vi "test_MonoMoveAndGetSlitPositionInMM.vi"(0 "device selection":enum16{"monochromator", "CCD", "SCD"}(ring), 1 "Test should pass":bool=TRUE, 5 "set-up a connection":bool=TRUE, 9 "tear down connection":bool=TRUE, 11 "error in":errorcluster, 12 "Delay between send and receive [ms]":i32=100, 13 "wait for procedure to be finished [ms]":i32=4000) -> (10 "log-file path":path, 15 "error out":errorcluster)   [LabVIEW 2023]
uses:
  Classes/Mono/Monochromator.lvclass
  <vilib>/addons/_JKI Toolkits/Caraya/classes/Assert/Assert Equal Value and Type_Variant.vi
  <vilib>/addons/_JKI Toolkits/Caraya/classes/Assert/Assert Not Error.vi
  <vilib>/addons/_JKI Toolkits/Caraya/classes/Test/Test.lvclass
  <vilib>/addons/_JKI Toolkits/Caraya/classes/Assert/Assert.lvclass
  <vilib>/Hampel Software Engineering/HSE Logger/hse-logger.lvlib
panel:
  out "device is open?":bool
  # "Connector Pane"
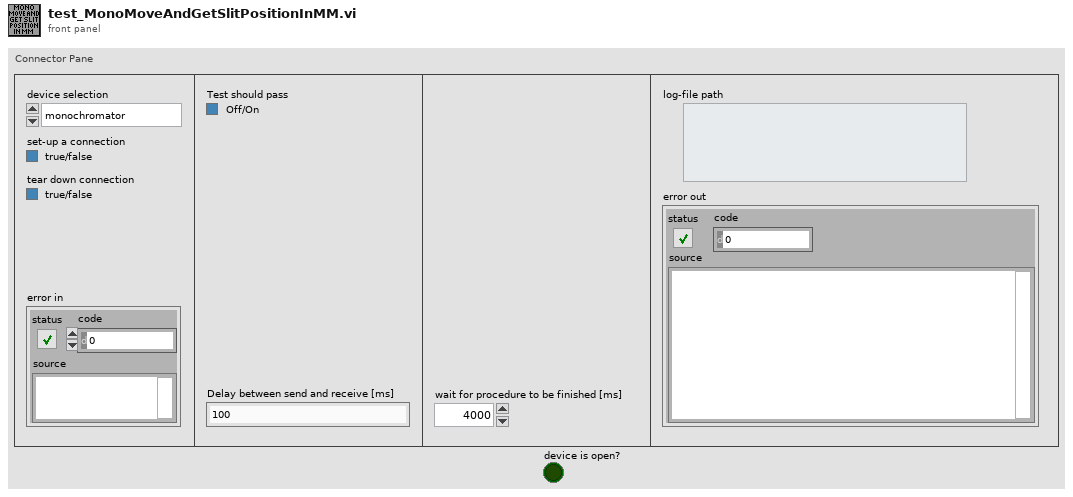
[diagram p1: front panel]
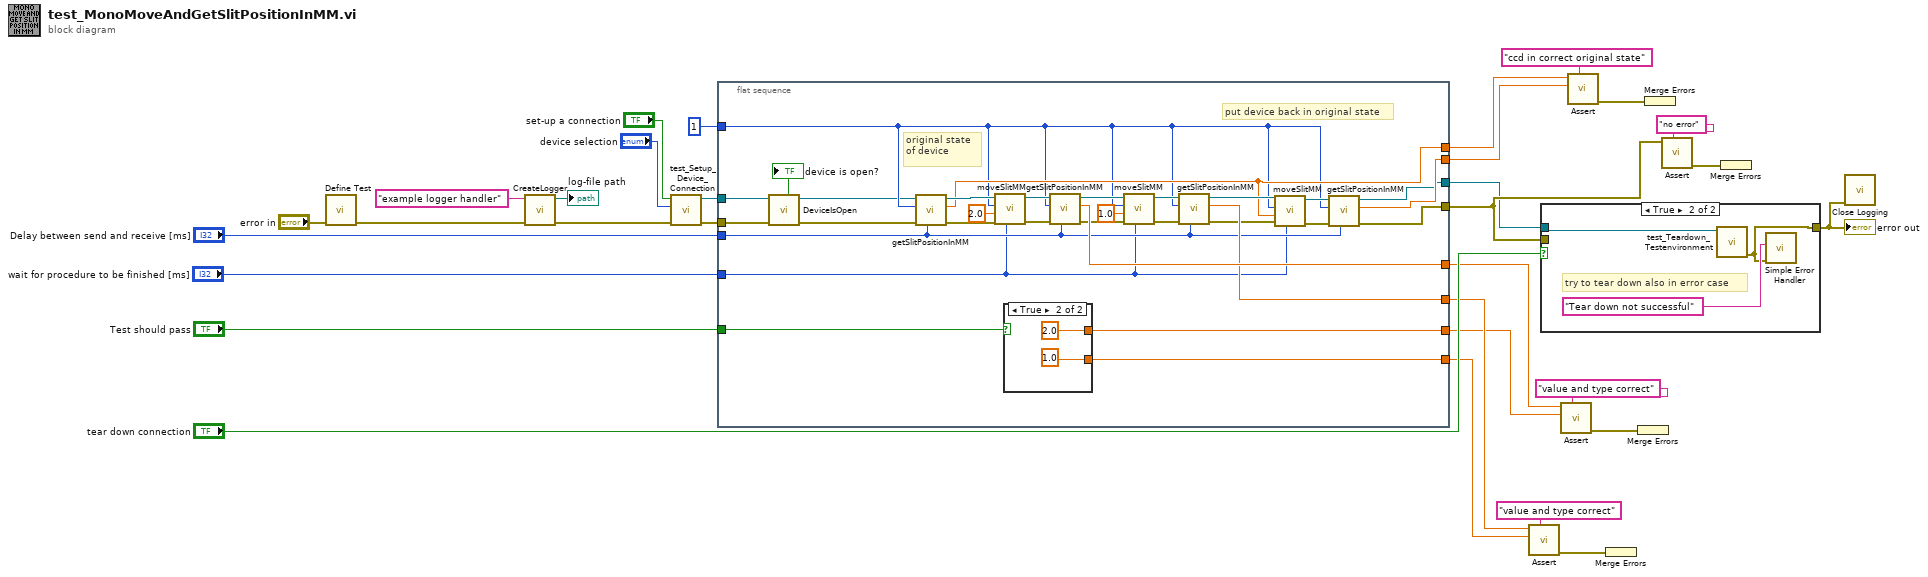
[diagram p0: block diagram]
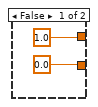
[diagram p2: hidden frame]
diagram:
  n1 = call <vilib>:"Define Test.vi"("error in (no error)"="error in") -> ("error out"=w4:errorcluster)  [unwired: 9 in, 1 out]
  n2 = call "CreateLogger.vi"("error in (no error)"=w4, "Handler Name"="example logger handler") -> ("error out"=w3:errorcluster, "log-file path"=→"log-file path":path)  [unwired: 8 in]
  n3 = call "test_Setup_Device_Connection.vi"("error in (no error)"=w3, "device selection"="device selection", "set-up a connection"="set-up a connection") -> ("error out"=w10:errorcluster, "Monochromator.lvclass"=w8:refnum<class "Monochromator.lvclass">)  [unwired: 5 in, 2 out]
  n4 = flat-sequence {
    tunnel: w10 -> [w33]
    tunnel: w8 -> [w35]
    tunnel: [w43] -> w22
    tunnel: "Test should pass" -> [w62]
    tunnel: [w44] -> w21
    tunnel: [w50] -> w20
    tunnel: [w61] -> w19
    tunnel: [w55] -> w18
    tunnel: [w60] -> w17
    tunnel: [w40] -> w14
    tunnel: [w45] -> w13
    tunnel: "Delay between send and receive [ms]" -> [w42]
    tunnel: "wait for procedure to be finished [ms]" -> [w41]
    tunnel: 1 ("type") -> [w38]
    frame #0 {
      # "put device back in original state"
      # "original state of device"
      n5 = call-dynamic "DeviceIsOpen.vi"("error in (no error)"=w33, "Monochromator in"=w35) -> ("error out"=w34:errorcluster, "device is open?"=→"device is open?":bool, "Monochromator out"=w36:refnum<class "Monochromator.lvclass">)  [unwired: 6 in, 1 out]
      n6 = call "getSlitPositionInMM.vi"("Delay between send and receive [ms]"=w42, "error in (no error)"=w34, "id"=w38, "Monochromator in"=w36) -> ("error out"=w58:errorcluster, "position"=w40:dbl, "Monochromator out"=w59:refnum<class "Monochromator.lvclass">)  [unwired: 5 in]
      n7 = call "moveSlitMM.vi"("Delay between send and receive [ms]"=w41, "error in (no error)"=w58, "position"=2.0, "id"=w38, "Monochromator in"=w59) -> ("error out"=w57:errorcluster, "Monochromator out"=w56:refnum<class "Monochromator.lvclass">)  [unwired: 3 in, 2 out]
      n8 = case shown="True" w62 {
        tunnel: [0.0 ("position") 1.0 ("position")] -> w61
        tunnel: [1.0 ("position") 2.0 ("position")] -> w60
        frame False {
        }
        frame True {
        }
      }
      n9 = call "getSlitPositionInMM.vi"("Delay between send and receive [ms]"=w42, "error in (no error)"=w57, "id"=w38, "Monochromator in"=w56) -> ("error out"=w51:errorcluster, "position"=w55:dbl, "Monochromator out"=w52:refnum<class "Monochromator.lvclass">)  [unwired: 5 in]
      n10 = call "moveSlitMM.vi"("Delay between send and receive [ms]"=w41, "error in (no error)"=w51, "position"=1.0, "id"=w38, "Monochromator in"=w52) -> ("error out"=w54:errorcluster, "Monochromator out"=w53:refnum<class "Monochromator.lvclass">)  [unwired: 3 in, 2 out]
      n11 = call "getSlitPositionInMM.vi"("Delay between send and receive [ms]"=w42, "error in (no error)"=w54, "id"=w38, "Monochromator in"=w53) -> ("error out"=w47:errorcluster, "position"=w50:dbl, "Monochromator out"=w48:refnum<class "Monochromator.lvclass">)  [unwired: 5 in]
      n12 = call "moveSlitMM.vi"("Delay between send and receive [ms]"=w41, "error in (no error)"=w47, "position"=w40, "id"=w38, "Monochromator in"=w48) -> ("error out"=w49:errorcluster, "Monochromator out"=w46:refnum<class "Monochromator.lvclass">)  [unwired: 3 in, 2 out]
      n13 = call "getSlitPositionInMM.vi"("Delay between send and receive [ms]"=w42, "error in (no error)"=w49, "id"=w38, "Monochromator in"=w46) -> ("error out"=w43:errorcluster, "position"=w45:dbl, "Monochromator out"=w44:refnum<class "Monochromator.lvclass">)  [unwired: 5 in]
    }
  }
  n14 = call-poly <vilib>:"Assert.vi"("Label"="value and type correct" ("Label (VI Title)"), "Y"=w19, "X"=w20) -> ("error out"=w30:errorcluster)  [unwired: 7 in, 1 out]
  n15 = case shown="True" "tear down connection" {
    tunnel: w21 -> [_ w69]
    tunnel: [w67 w68] -> w1
    tunnel: w22 -> [w67 _]
    frame False {
    }
    frame True {
      # "try to tear down also in error case"
      n16 = call "test_Teardown_Testenvironment.vi"("GenericDevice.lvclass"=w69) -> ("error out"=w68:errorcluster)  [unwired: 9 in, 1 out]
      n17 = call <vilib>:"Simple Error Handler.vi"("error source (\" \")"="Tear down not successful" ("error source (\" \")"), "error in (no error)"=w68) -> ()  [unwired: 3 in, 5 out]
    }
  }
  "error out" <- w1
  n18 = call-poly <vilib>:"Assert.vi"("Label"="value and type correct" ("Label (VI Title)"), "Y"=w17, "X"=w18) -> ("error out"=w29:errorcluster)  [unwired: 7 in, 1 out]
  n19 = call-poly <vilib>:"Assert.vi"("Label"="ccd in correct original state" ("Label (VI Title)"), "Y"=w13, "X"=w14) -> ("error out"=w16:errorcluster)  [unwired: 7 in, 1 out]
  n20 = Merge Errors(w30) -> ()  [unwired: 1 out]
  n21 = Merge Errors(w29) -> ()  [unwired: 1 out]
  n22 = Merge Errors(w16) -> ()  [unwired: 1 out]
  n23 = call-poly <vilib>:"Assert.vi"("Label"="no error" ("Label (VI Title)"), "Not Error?"=w22) -> ("error out"=w24:errorcluster)  [unwired: 8 in, 1 out]
  n24 = Merge Errors(w24) -> ()  [unwired: 1 out]
  n25 = call <vilib>:"Close Logging.vi"("error in"=w1) -> ()  [unwired: 10 in, 1 out]
